vi "RequiredLinkBudget.vi"(2 "Bandwith (MHz)":dbl, 3 "Bit rate (bits/s)":dbl, 4 "Chosen Modulation":string(combo)) -> (0 "C/N (dB) required":dbl, 1 "C/N0 (dB) required":dbl)   [LabVIEW 2015]
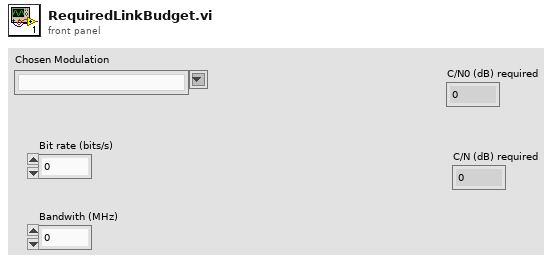
[diagram p1: front panel]
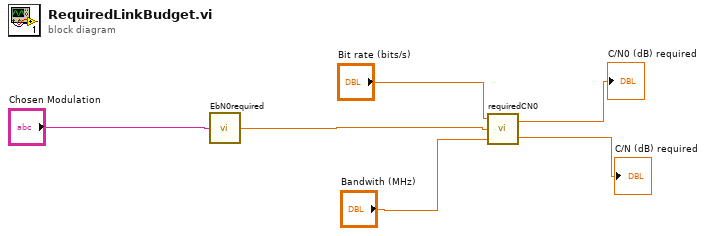
[diagram p0: block diagram]
diagram:
  n1 = call "EbN0required.vi"("Modulation"="Chosen Modulation") -> ("Eb/N0 (dB) required for BER=10-4"=w5:dbl)
  n2 = call "requiredCN0.vi"("Channel Bandwith (MHz)"="Bandwith (MHz)", "Eb/N0 required (dB)"=w5, "Bit rate (bits/s)"="Bit rate (bits/s)") -> ("C/N required (dB)"=→"C/N (dB) required":dbl, "C/N0 required (dB)"=→"C/N0 (dB) required":dbl)
